vi "lab1_Shimeng_LI.vi"() -> ()   [LabVIEW 2014]
uses:
  <vilib>/Utility/file.llb/Read From Spreadsheet File (DBL).vi
  <vilib>/imath/engines/lvmath2/RunTimeEngine/ArithmeticOperatorToken/NIMS_ArithmeticOperator_plus.vi
  <instcachedir>/0/NIMS_ArithmeticOperator_plus_48D6EAACA5D645B09F7EC9C016C2DEA8.lvgen/NIMS_ArithmeticOperator_plus_48D6EAACA5D645B09F7EC9C016C2DEA8_004.vi
  <vilib>/imathl/engines/lvmath/Functions/Error Handling/Create Error.vi
  <vilib>/imath/engines/lvmath2/RunTimeEngine/ArithmeticOperatorToken/NIMS_ArithmeticOperator_minus.vi
  <instcachedir>/0/NIMS_ArithmeticOperator_minus_39C0593E74DA4138ACA2AB742906488D.lvgen/NIMS_ArithmeticOperator_minus_39C0593E74DA4138ACA2AB742906488D_003.vi
  <vilib>/imath/engines/lvmath2/RunTimeEngine/NodeEndStatement/NIMS_NodeEndStatement_Output.vi
  <instcachedir>/0/NIMS_NodeEndStatement_Output_53EC0D466D134D7ABD903AC30B43404B.lvgen/NIMS_NodeEndStatement_Output_53EC0D466D134D7ABD903AC30B43404B_005.vi
  <vilib>/imath/engines/lvmath2/RunTimeEngine/ErrorHandling/NIMS_Finalize Error.vi
panel:
  out "o":dbl
  out "a":dbl
  out "Y0":dbl
  out "X0":dbl
  out "new y":dbl[](array[numeric])
  out "new x":dbl[](array[numeric])
  out "global y":dbl[](array[numeric])
  out "global x":dbl[](array[numeric])
  out "local y":dbl[](array[numeric])
  out "local x":dbl[](array[numeric])
  out "New Object Points Global":dbl[][](array[numeric])
  out "New  point":dbl[][](array[numeric]) format="%0.3f"
  in  "file path of new point":path
  out "local coordinates":dbl[][](array[numeric]) format="%0.3f"
  in  "file path of local coordinates":path
  out "resY":dbl[](array[numeric])
  out "resX":dbl[](array[numeric])
  out "Global Coordinates":dbl[][](array[numeric]) format="%0.3f"
  in  "file path of global coordinates":path
  # "Helmert  Transformation"
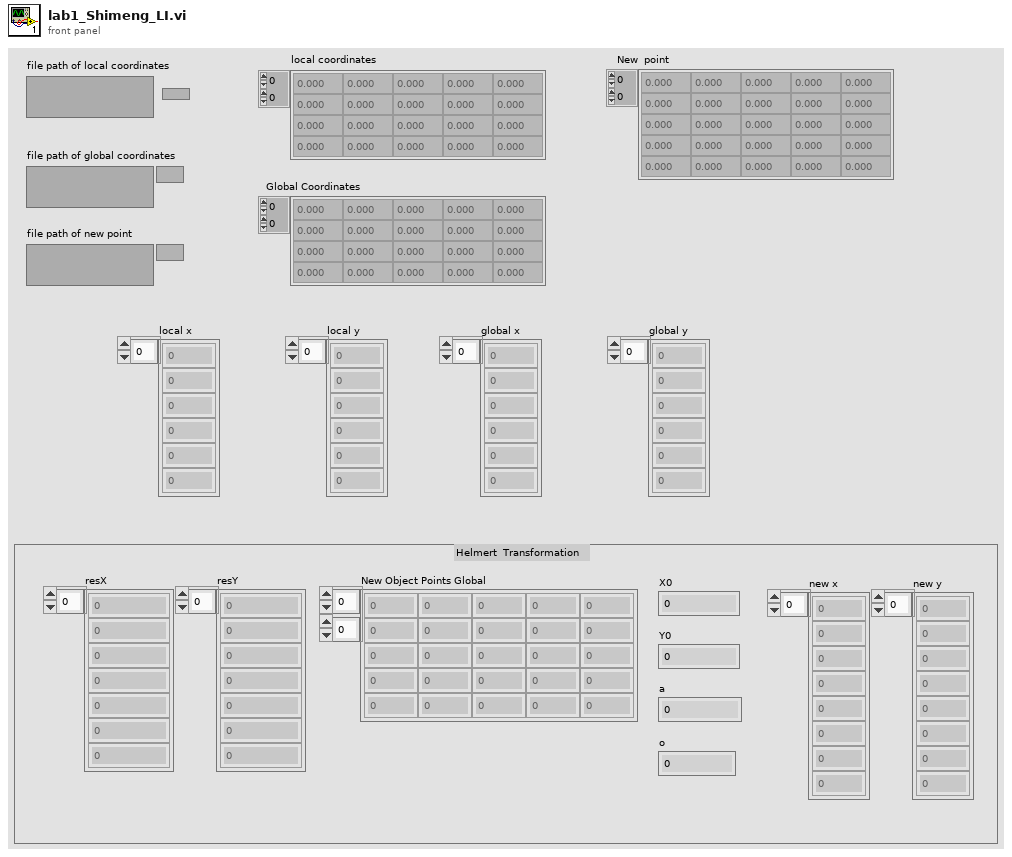
[diagram p1: front panel]
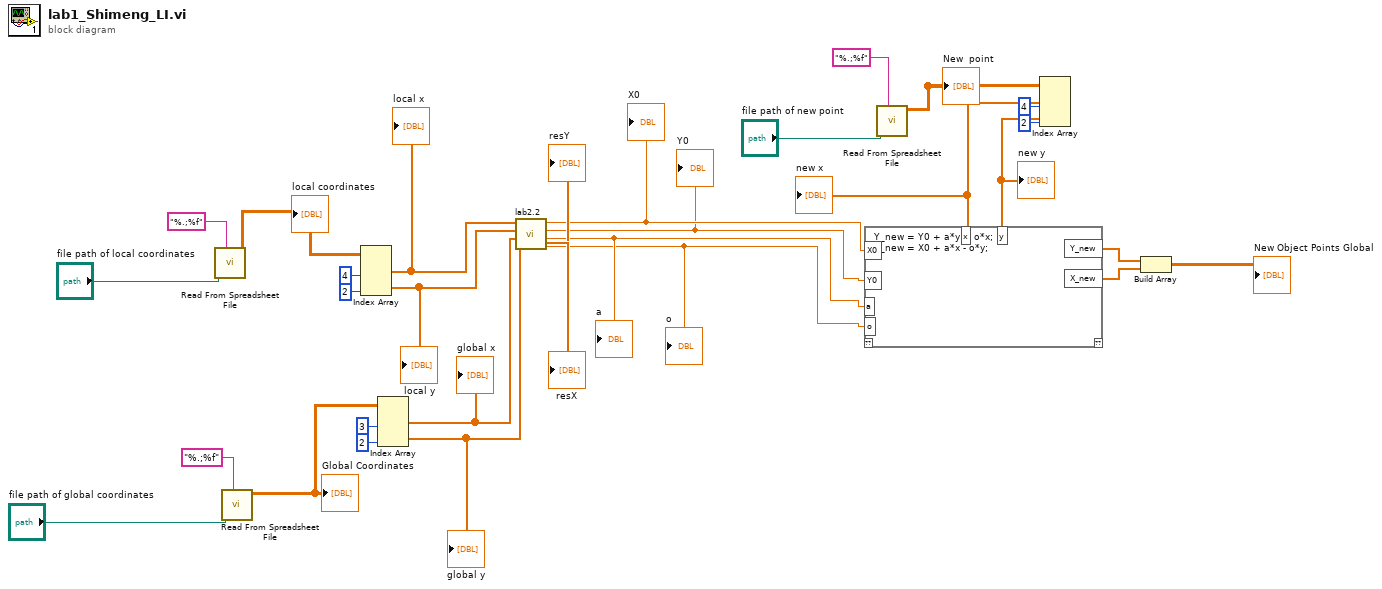
[diagram p0: block diagram]
diagram:
  n1 = call-poly <vilib>:"Read From Spreadsheet File.vi"("format (%.3f)"="%.;%f", "file path (dialog if empty)"="file path of local coordinates") -> ("all rows"=w17:dbl[][])  [unwired: 5 in, 4 out]
  "local coordinates" <- w17
  n2 = call-poly <vilib>:"Read From Spreadsheet File.vi"("format (%.3f)"="%.;%f", "file path (dialog if empty)"="file path of global coordinates") -> ("all rows"=w29:dbl[][])  [unwired: 5 in, 4 out]
  "Global Coordinates" <- w29
  n3 = Index Array(array=w17, index (col) #1=4 ("index (col)"), index (col) #2=2 ("index (col)")) -> (element #1=w24:dbl[], element #2=w23:dbl[])  [unwired: 2 in]
  "local x" <- w24
  "local y" <- w23
  n4 = Index Array(array=w29, index (col) #1=3 ("disabled index (col)"), index (col) #2=2 ("disabled index (col)")) -> (element #1=w26:dbl[], element #2=w25:dbl[])  [unwired: 2 in]
  "global x" <- w26
  "global y" <- w25
  n5 = call "lab2.2.vi"("y global"=w25, "x global"=w26, "y local"=w23, "x local"=w24) -> ("o"=w11:dbl, "a"=w12:dbl, "Y0"=w13:dbl, "X0"=w14:dbl, "resY"=→"resY":dbl[], "resX"=→"resX":dbl[])  [unwired: 2 in]
  "X0" <- w14
  "Y0" <- w13
  "a" <- w12
  "o" <- w11
  n6 = call-poly <vilib>:"Read From Spreadsheet File.vi"("format (%.3f)"="%.;%f", "file path (dialog if empty)"="file path of new point") -> ("all rows"=w9:dbl[][])  [unwired: 5 in, 4 out]
  "New  point" <- w9
  n7 = Index Array(array=w9, index (col) #1=4 ("disabled index (col)"), index (col) #2=2 ("index (col)")) -> (element #1=w6:dbl[], element #2=w5:dbl[])  [unwired: 2 in]
  "new x" <- w6
  "new y" <- w5
  n8 = mathscript code="Y_new = Y0 + a*y + o*x;\nX_new = X0 + a*x - o*y;"("X0"=w14, "Y0"=w13, "a"=w12, "o"=w11, "x"=w6, "y"=w5) -> ("Y_new"=w16:dbl[], "X_new"=w15:dbl[])  [unwired: 1 in, 1 out]
  n9 = Build Array(w16, w15) -> (→"New Object Points Global":dbl[][])
